vi "flattenToString.vi"(8 "error in (no error)":errorcluster, 11 "Worker Status in":refnum<class "Worker Status.lvclass">) -> (0 "error out":errorcluster, 3 "data string":string)   [LabVIEW 2017, in "Message Interface.lvlib" / "Worker Status.lvclass"]
uses:
  Worker Status.lvclass
  C:/Users/Public/Documents/wc/BuildFarm/src/LabVIEW/vi.lib/BenjaminR/Build Farm/Classes/Message Interface/Status/Status.lvclass
  Status/Status.lvclass/Status.ctl
  Status/Read Item Name.vi
  Status/Write Item Name.vi
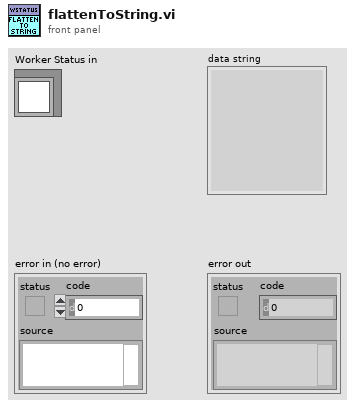
[diagram p1: front panel]
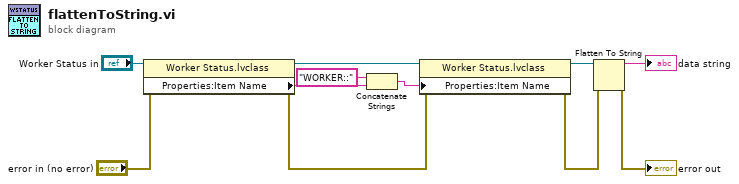
[diagram p0: block diagram]
diagram:
  n1 = property class="Worker Status.lvclass"(reference="Worker Status in", error in="error in (no error)") -> (reference out=w10:refnum<class "Worker Status.lvclass">, error out=w9:errorcluster, "Properties:Item Name"=w6:string)
  n2 = Concatenate Strings("WORKER::" ("string"), w6) -> (w7:string)
  n3 = property class="Worker Status.lvclass"(reference=w10, error in=w9, "Properties:Item Name"=w7) -> (reference out=w4:refnum<class "Worker Status.lvclass">, error out=w1:errorcluster)
  n4 = Flatten To String(anything=w4, error in (no error)=w1) -> (data string=→"data string":string, error out=→"error out":errorcluster)  [unwired: 2 in, 1 out]
